vi "Error handler.vi"() -> (3 "Enum":T1)   [LabVIEW 2020]
uses:
  Estados.ctl
  Variables Globales.vi
panel:
  in  "Modo Manual":bool
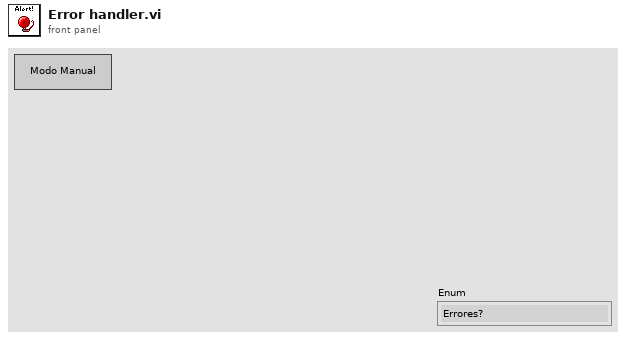
[diagram p1: front panel]
types:
  T1 = typedef "Estados.ctl" = enum16{"Errores?", "Modo Manual?", "Control de válvula alt.", "Control de válvula", "Nivel bajo?", "Query nivel del tanque", "Query peso del pote", "Ajuste?", "Llenado?", "Emergencia?", "Init", "Ajuste", "Nivel Bajo", "Llenado", "Error", "Emergencia"}
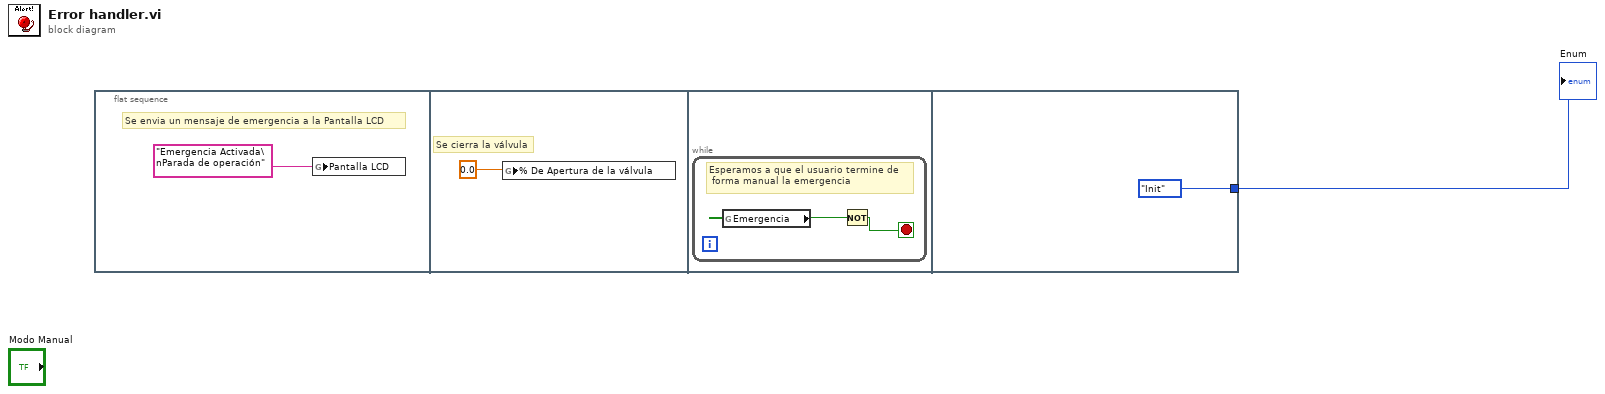
[diagram p0: block diagram]
diagram:
  n1 = flat-sequence {
    tunnel: [Estados."Init"] -> w1
    frame #0 {
      # "Se envia un mensaje de emergencia a la Pantalla LCD"
      n2 = global write "Variables Globales.vi" "Pantalla LCD"("Emergencia Activada\nParada de operación") -> ()
    }
    frame #1 {
      # "Se cierra la válvula"
      n3 = global write "Variables Globales.vi" "% De Apertura de la válvula"(0.0) -> ()
    }
    frame #2 {
      n4 = while {
        stop <- w4 stop-if-true
        # "Esperamos a que el usuario termine de\n forma manual la emergencia"
        n5 = global read "Variables Globales.vi" "Emergencia"() -> (w5:bool)
        n6 = Not(x=w5) -> (.not. x?=w4:bool)
      }
    }
    frame #3 {
    }
  }
  "Enum" <- w1
